vi "Resistance2Temperature.vi"(8 "Pt Type":T1, 10 "Actual resistance":dbl) -> (2 "Pt temperature":dbl)   [LabVIEW 2022 SP3]
uses:
  controls/Pt_type.ctl
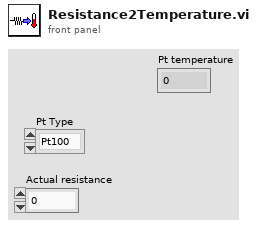
[diagram p1: front panel]
types:
  T1 = typedef "Pt_type.ctl" = enum16{"Pt100", "Pt1000"}
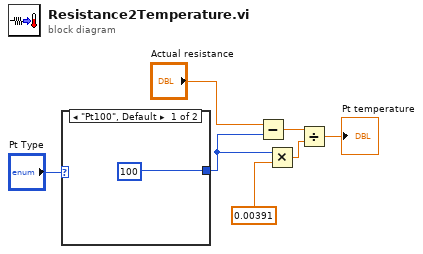
[diagram p0: block diagram]
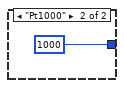
[diagram p2: hidden frame]
diagram:
  n1 = case shown="\"Pt100\", Default" "Pt Type" {
    tunnel: [100 1000] -> w3
    frame "Pt100", Default {
    }
    frame "Pt1000" {
    }
  }
  n2 = Subtract(x="Actual resistance", y=w3) -> (x-y=w5:dbl)
  n3 = Multiply(x=w3, y=0.00391) -> (x*y=w4:dbl)
  n4 = Divide(x=w5, y=w4) -> (x/y=→"Pt temperature":dbl)
